vi "Get BandLimits.vi"(4 "error in (no error)":errorcluster, 7 "VISA resource name":refnum<visa-resource-name>) -> (0 "error out":errorcluster, 1 "LowerBand (out)":dbl min=-100.0 max=0.0, 2 "UpperBand (out)":dbl=100.0 max=100.0, 3 "VISA resource name out":refnum<visa-resource-name>)   [LabVIEW 2015, in "JULABO DeviceDriver.lvlib"]
doc: "This VI returns the maximum allowed difference between internal and external temperature during heating up and cooling down.\n\nNote:\nThis function is not available for instruments which do not support different values for upper and lower bandlimit. Please use <B>JULABO_Configure_GetBand.vi</B> in case your instrument supports only one bandlimit. See operating manual to check whether your instrument supports different values for lower and upper bandlimit.\n\nThis function is not available for devices which does not have an external sensor plug."
uses:
  JULABO DeviceDriver.lvlib
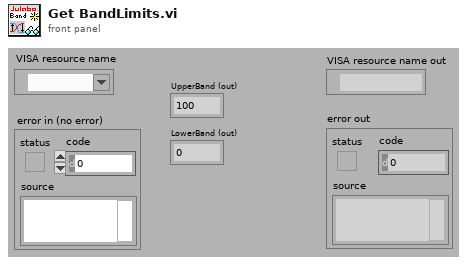
[diagram p1: front panel]
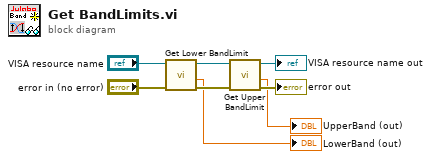
[diagram p0: block diagram]
diagram:
  n1 = call "Get Lower BandLimit.vi"("error in (no error)"="error in (no error)", "VISA resource name"="VISA resource name") -> ("error out"=w5:errorcluster, "LowerBand (out)"=→"LowerBand (out)":dbl, "VISA resource name out"=w6:refnum<visa-resource-name>)  [unwired: 7 in]
  n2 = call "Get Upper BandLimit.vi"("error in (no error)"=w5, "VISA resource name"=w6) -> ("error out"=→"error out":errorcluster, "UpperBand (out)"=→"UpperBand (out)":dbl, "VISA resource name out"=→"VISA resource name out":refnum<visa-resource-name>)  [unwired: 7 in]
